vi "PH_uOPA_DelayController.ProcCases.vi"(0 "i ref in":refnum<vi>, 1 "selector":string, 2 "Data":T1, 3 "call cluster":T2={"Object"="", "Selector"="", "CallType"=enum."synchronous", "Async Object"="", "Async Selector"="", "Data Descriptor"="", "Data"=[], "Error #"=0, "Expire"=0}, 5 "error in (no error)":errorcluster) -> (14 "i ref out":refnum<vi>, 17 "answer cluster":T2={"Object"="", "Selector"="", "CallType"=enum."synchronous", "Async Object"="", "Async Selector"="", "Data Descriptor"="", "Data"=[], "Error #"=0, "Expire"=0}, 19 "error out":errorcluster)   [LabVIEW 2014, in "PH_uOPA_DelayController.lvlib"]
doc: "This method is called by a process from within the default case in the event loop. The methods of a class that are linked to events will be called from THIS method. Add your code here."
uses:
  PH_uOPA_DelayController.lvlib
  CS_Core/CSSystem/CoreDefs/CoreDefs.call_type.ctl
  CS_Core/BaseProcess/BaseProcess.descriptor string definition.ctl
  CS_Core/CSSystem/CoreDefs/CoreDefs.rawDataType.ctl
  PH_Basics/PH_StatusHandler/PH_StatusHandler.Status.ctl
  PH_uOPA_DelayController.Limit.ctl
  CS_Core/CSSystem/CoreLib/CoreLib.string 2 byte array.vi
  CS_Core/CSSystem/CoreLib/CoreLib.byte array 2 double.vi
  CS_Core/CSSystem/CoreLib/CoreLib.byte array 2 int.vi
  CS_Core/CSSystem/CoreLib/CoreLib.byte array 2 short.vi
  CS_Core/BaseProcess/BaseProcess.lvlib
  CS_Core/CSSystem/CoreLib/CoreLib.lvlib
  CS_Core/CAEObj/CAEObj.lvlib
  PH_Basics/PH_PSDBWriter/PH_PSDBWriter.lvlib
  PH_Devices/PH_TKTDS-30xx/PH_TKTDS-30xx.lvlib
  PH_Basics/PH_StatusHandler/PH_StatusHandler.lvlib
  PH_Basics/PH_AxisGUI_BaseClass/PH_AxisGUI_BaseClass.lvlib
  PH_Basics/PH_Stepmotor_BaseClass/PH_Stepmotor_BaseClass.lvlib
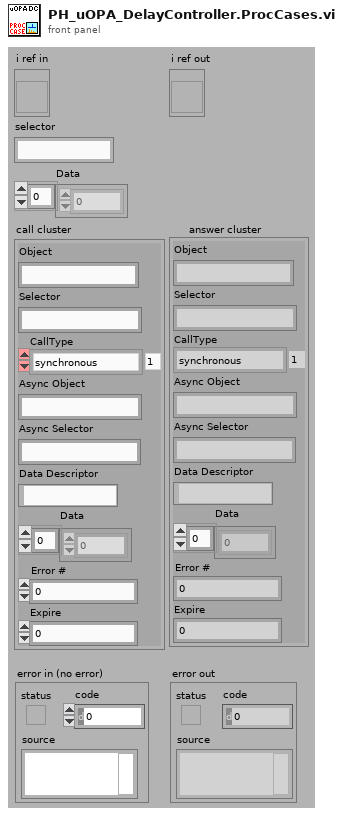
[diagram p1: front panel]
types:
  T1 = typedef "CoreDefs.rawDataType.ctl" = i8[]
  T2 = typedef "CoreDefs.call_type.ctl" = cluster{"Object":string, "Selector":string, "CallType":enum16{"simple", "synchronous", "asynchronous"}, "Async Object":string, "Async Selector":string, "Data Descriptor":T3, "Data":T1, "Error #":i32, "Expire":u32}
  T3 = typedef "BaseProcess.lvlib/BaseProcess.descriptor string definition.ctl" = string
  T4 = typedef "PH_uOPA_DelayController.lvlib/PH_uOPA_DelayController.Limit.ctl" = cluster{"low":dbl, "activate":dbl, "fine":dbl}
  T5 = typedef "PH_StatusHandler.lvlib/PH_StatusHandler.Status.ctl" = i16
  T6 = typedef "PH_PSDBWriter.lvlib/PH_PSDBWriter.PHELIX-Subsystems.ctl" = i32
  T7 = typedef "PH_Stepmotor_BaseClass.lvlib/PH_Stepmotor_BaseClass.Axis Settings.ctl" = cluster{"Sign change":bool, "Width":dbl, "Calibration":dbl, "Unit":string, "Motor Type":T8, "Unit Width":string, "Unit CF":string}
  T8 = typedef "PH_Stepmotor_BaseClass.lvlib/PH_Stepmotor_BaseClass.Motor Type.ctl" = enum16{"Unspecific", "OWIS 49.120.2633", "OWIS 49.060.1033", "OWIS 43.040.2558", "Diamond Motion 2200 series", "OWIS 49.120.266B.MV6", "Calorimeter", "Linear Stage 1", "MICOS VT-80", "MICOS VT-80 S", "Standa Rotstage nt0.95A", "PUF RA 320.200", "PUF RA 800.200", "PUF RA 800.400", "PUF RA 400.50", "1324.nn.800.50", "1324.n9c.800.50", "1324.nn.320.200", "1324.nn.400.200", "1324.nn.800.200", "1324.nn.400.50", "1324.8c9c.800.50", "1324.8c9c.400.200"}
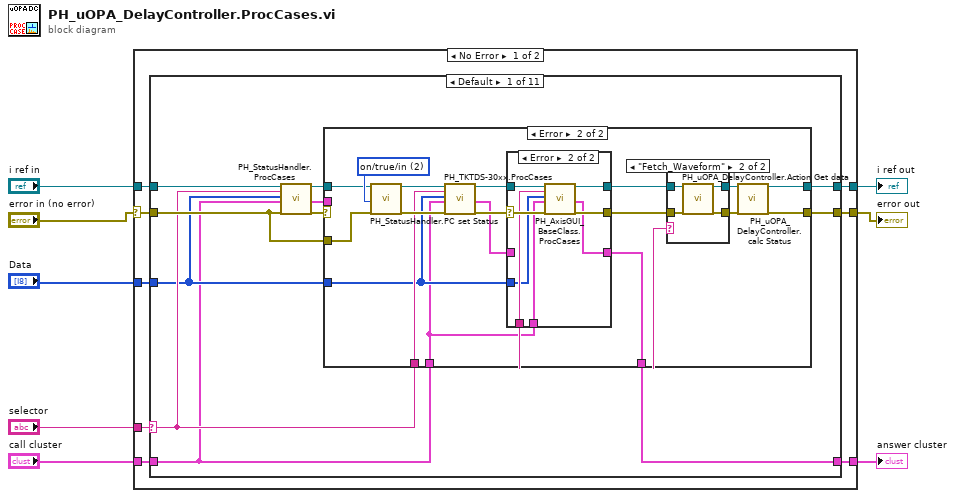
[diagram p0: block diagram]
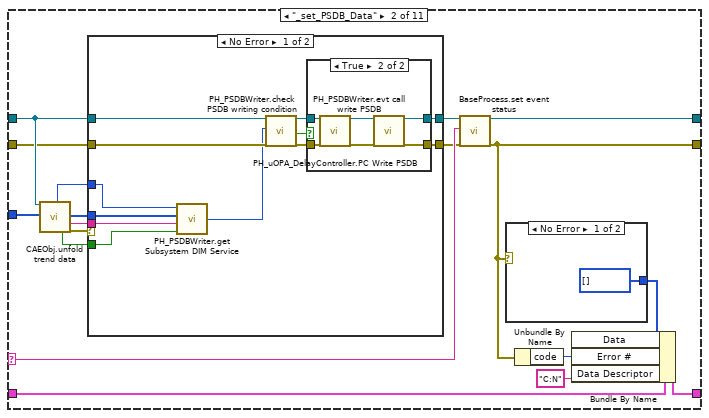
[diagram p5: hidden frame]
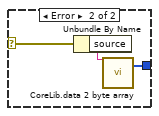
[diagram p8: hidden frame]
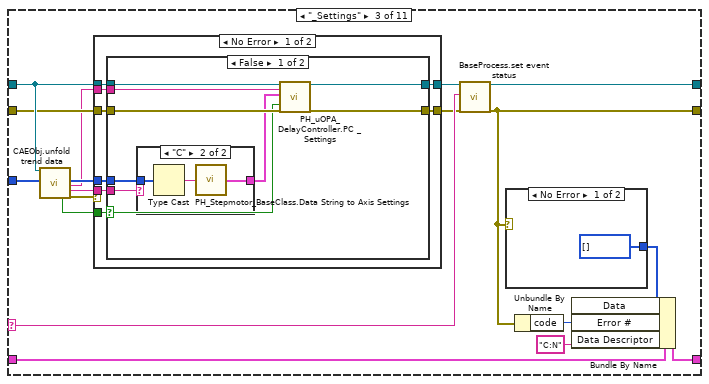
[diagram p9: hidden frame]
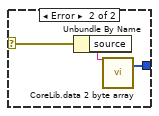
[diagram p13: hidden frame]
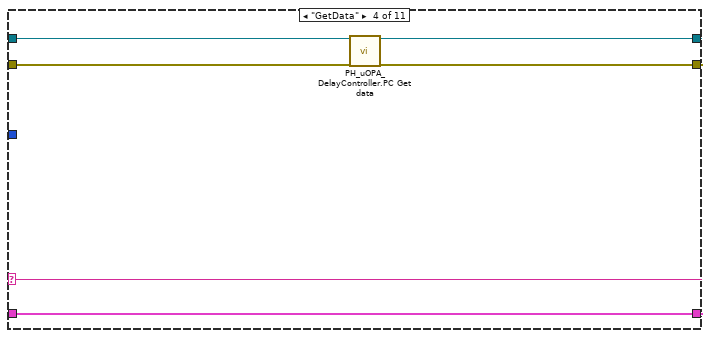
[diagram p14: hidden frame]
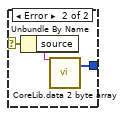
[diagram p15: hidden frame]
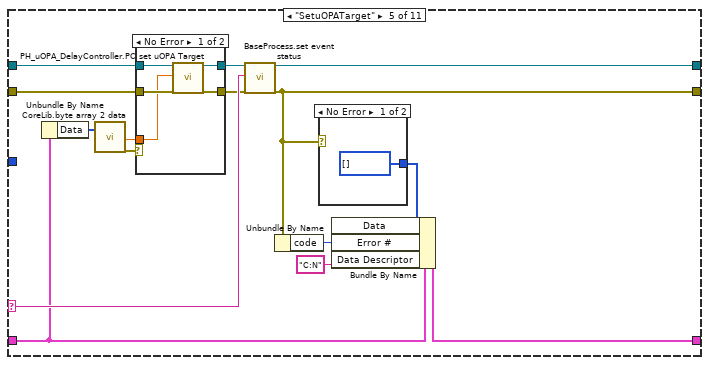
[diagram p16: hidden frame]
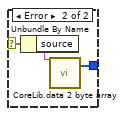
[diagram p18: hidden frame]
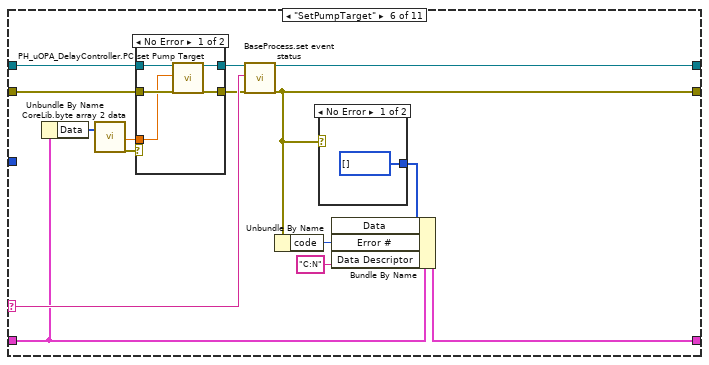
[diagram p19: hidden frame]
diagram:
  n1 = case shown="No Error" "error in (no error)" {
    selector: "error in (no error)" -> [w9 w369]
    tunnel: "selector" -> [w16 _]
    tunnel: [w15 w370] -> w7
    tunnel: "Data" -> [w14 _]
    tunnel: "call cluster" -> [w13 w370]
    tunnel: "i ref in" -> [w12 w371]
    tunnel: [w11 w371] -> w3
    tunnel: [w10 w369] -> w2
    frame No Error {
      n2 = case shown="Default" w16 {
        selector: w16 -> [w19 w78 w122 w161 w181 w207 w233 w259 w287 w316 w348]
        tunnel: w14 -> [w18 w66 w119 _ _ _ _ _ _ _ _]
        tunnel: w12 -> [w24 w70 w118 w159 w176 w202 w228 w254 w282 w311 w343]
        tunnel: [w27 w77 w121 w163 w172 w198 w224 w250 w278 w307 w333] -> w11
        tunnel: w13 -> [w17 w82 w126 w160 w179 w205 w231 w257 w285 w314 w346]
        tunnel: [w25 w81 w125 w166 w185 w211 w237 w263 w291 w320 w352] -> w15
        tunnel: w9 -> [w22 w68 w116 w158 w180 w206 w232 w258 w286 w315 w347]
        tunnel: [w26 w79 w123 w164 w183 w209 w235 w261 w289 w318 w350] -> w10
        frame Default {
          n3 = call "PH_StatusHandler.ProcCases.vi"("i ref in"=w24, "selector"=w19, "Data"=w18, "call cluster"=w17, "error in (no error)"=w22) -> ("i ref out"=w23:refnum<vi>, "answer cluster"=w20:T2, "error out"=w21:errorcluster)  [unwired: 12 in]
          n4 = case shown="Error" w21 {
            selector: w21 -> [w29 _]
            tunnel: [w30 w45] -> w27
            tunnel: [w29 w44] -> w26
            tunnel: w19 -> [_ w37]
            tunnel: w18 -> [_ w36]
            tunnel: w17 -> [_ w35]
            tunnel: [w28 w33] -> w25
            tunnel: w22 -> [_ w32]
            tunnel: w23 -> [w30 w31]
            tunnel: w20 -> [w28 _]
            frame No Error {
            }
            frame Error {
              w48 = T5 2 items=["no info", "off/false/out", "on/true/in", "Failure", "Alarm", "Status 1", "Status 2", "Status 3"] ("Status")
              n5 = call "PH_StatusHandler.PC set Status.vi"("i ref in"=w31, "Status"=w48, "error in (no error)"=w32) -> ("i ref out"=w47:refnum<vi>, "error out"=w46:errorcluster)  [unwired: 15 in]
              n6 = call "PH_TKTDS-30xx.ProcCases.vi"("i ref in"=w47, "selector"=w37, "Data"=w36, "call cluster"=w35, "error in (no error)"=w46) -> ("i ref out"=w40:refnum<vi>, "answer cluster"=w34:T2, "error out"=w38:errorcluster)  [unwired: 12 in]
              n7 = case shown="Error" w38 {
                selector: w38 -> [w50 w56]
                tunnel: [w50 w59] -> w41
                tunnel: w40 -> [w51 w58]
                tunnel: [w51 w57] -> w39
                tunnel: w37 -> [_ w55]
                tunnel: w36 -> [_ w54]
                tunnel: w35 -> [_ w53]
                tunnel: [w49 w52] -> w33
                tunnel: w34 -> [w49 _]
                frame No Error {
                }
                frame Error {
                  n8 = call "PH_AxisGUI_BaseClass.ProcCases.vi"("i ref in"=w58, "selector"=w55, "data"=w54, "call cluster"=w53, "error in"=w56) -> ("i ref out"=w57:refnum<vi>, "answer cluster"=w52:T2, "error out"=w59:errorcluster)  [unwired: 12 in]
                }
              }
              n9 = case shown="\"Fetch_Waveform\"" w37 {
                tunnel: w39 -> [w61 w65]
                tunnel: [w61 w64] -> w43
                tunnel: w41 -> [w60 w63]
                tunnel: [w60 w62] -> w42
                frame Default {
                }
                frame "Fetch_Waveform" {
                  n10 = call "PH_uOPA_DelayController.Action Get data.vi"("i ref in"=w65, "error IO"=w63) -> ("i ref out"=w64:refnum<vi>, "error out"=w62:errorcluster)  [unwired: 16 in]
                }
              }
              n11 = call "PH_uOPA_DelayController.calc Status.vi"("i ref in"=w43, "error in"=w42) -> ("i ref out"=w45:refnum<vi>, "error out"=w44:errorcluster)  [unwired: 16 in]
            }
          }
        }
        frame "_set_PSDB_Data" {
          n12 = call "CAEObj.unfold trend data.vi"("i ref in"=w70, "raw trend data"=w66) -> ("quality"=w71:i32, "no link"=w74:bool, "data"=w72:i8[], "typeDescriptor"=w73:string, "error out"=w75:errorcluster)  [unwired: 9 in, 4 out]
          n13 = case shown="No Error" w75 {
            tunnel: w68 -> [w95 w105]
            tunnel: [w94 w104] -> w69
            tunnel: [w93 w105] -> w67
            tunnel: w70 -> [w91 w104]
            tunnel: w74 -> [w86 _]
            tunnel: w73 -> [w87 _]
            tunnel: w72 -> [w88 _]
            tunnel: w71 -> [w85 _]
            frame No Error {
              n14 = call "PH_PSDBWriter.get Subsystem DIM Service.vi"("no link"=w86, "typeDescriptor"=w87, "data"=w88, "quality"=w85) -> ("PHELIX Subsystems"=w84:T6)
              n15 = call "PH_PSDBWriter.check PSDB writing condition.vi"("i ref in"=w91, "wanted Subsystem"=w84, "error IO"=w95) -> ("i ref out"=w90:refnum<vi>, "write PSDB?"=w89:bool, "error out"=w92:errorcluster)  [unwired: 14 in]
              n16 = case shown="True" w89 {
                tunnel: w92 -> [w96 w103]
                tunnel: [w97 w100] -> w94
                tunnel: [w96 w98] -> w93
                tunnel: w90 -> [w97 w102]
                frame False {
                }
                frame True {
                  n17 = call "PH_uOPA_DelayController.PC Write PSDB.vi"("i ref in"=w102, "error IO"=w103) -> ("i ref out"=w101:refnum<vi>, "error out"=w99:errorcluster)  [unwired: 16 in]
                  n18 = call "PH_PSDBWriter.evt call write PSDB.vi"("i ref in"=w101, "error in (no error)"=w99) -> ("i ref out"=w100:refnum<vi>, "error out"=w98:errorcluster)  [unwired: 16 in]
                }
              }
            }
            frame Error {
            }
          }
          n19 = call "BaseProcess.set event status.vi"("i ref in"=w69, "EventStatus"=w78, "error in (no error)"=w67) -> ("i ref out"=w77:refnum<vi>, "error out"=w79:errorcluster)  [unwired: 14 in, 1 out]
          n20 = case shown="No Error" w79 {
            selector: w79 -> [_ w109]
            tunnel: [T1 [] ("byteArray out") w108] -> w80
            frame No Error {
            }
            frame Error {
              n21 = Unbundle By Name(w109) -> ("source"=w107:string)
              n22 = call-poly "CoreLib.data 2 byte array.vi"("string"=w107) -> ("byteArray out"=w108:T1)  [unwired: 18 in]
            }
          }
          n23 = Unbundle By Name(w79) -> ("code"=w83:i32)
          n24 = Bundle By Name(cluster=w82, "Data"=w80, "Error #"=w83, "Data Descriptor"="C:N") -> (w81:T2)
        }
        frame "_Settings" {
          n25 = call "CAEObj.unfold trend data.vi"("i ref in"=w118, "raw trend data"=w119) -> ("no link"=w111:bool, "data"=w114:i8[], "serviceName"=w113:string, "typeDescriptor"=w110:string, "error out"=w112:errorcluster)  [unwired: 9 in, 4 out]
          n26 = case shown="No Error" w112 {
            tunnel: w114 -> [w130 _]
            tunnel: w118 -> [w134 w151]
            tunnel: [w133 w151] -> w117
            tunnel: w116 -> [w135 w150]
            tunnel: [w132 w150] -> w115
            tunnel: w111 -> [w131 _]
            tunnel: w110 -> [w129 _]
            tunnel: w113 -> [w128 _]
            frame No Error {
              n27 = case "NO LINK?" shown="False" w131 {
                selector: w131 -> [w141 _]
                tunnel: w135 -> [w143 w149]
                tunnel: w134 -> [w144 w148]
                tunnel: [w139 w148] -> w133
                tunnel: [w140 w149] -> w132
                tunnel: w129 -> [w137 _]
                tunnel: w130 -> [w138 _]
                tunnel: w128 -> [w142 _]
                frame False {
                  n28 = case shown="\"C\"" w137 {
                    tunnel: [_ w145] -> w136
                    tunnel: w138 -> [_ w147]
                    frame Default {
                    }
                    frame "C" {
                      n29 = Type Cast(x=w147) -> (*(type *) &x=w146:string)  [unwired: 1 in]
                      n30 = call "PH_Stepmotor_BaseClass.Data String to Axis Settings.vi"("Data String"=w146) -> ("Axis Settings"=w145:T7)  [unwired: 1 out]
                    }
                  }
                  n31 = call "PH_uOPA_DelayController.PC _Settings.vi"("VI in"=w144, "serviceName"=w142, "Axis Settings"=w136, "no link"=w141, "error in (no error)"=w143) -> ("VI out"=w139:refnum<vi>, "error out"=w140:errorcluster)  [unwired: 13 in]
                }
                frame True {
                }
              }
            }
            frame Error {
            }
          }
          n32 = call "BaseProcess.set event status.vi"("i ref in"=w117, "EventStatus"=w122, "error in (no error)"=w115) -> ("i ref out"=w121:refnum<vi>, "error out"=w123:errorcluster)  [unwired: 14 in, 1 out]
          n33 = case shown="No Error" w123 {
            selector: w123 -> [_ w155]
            tunnel: [T1 [] ("byteArray out") w154] -> w124
            frame No Error {
            }
            frame Error {
              n34 = Unbundle By Name(w155) -> ("source"=w153:string)
              n35 = call-poly "CoreLib.data 2 byte array.vi"("string"=w153) -> ("byteArray out"=w154:T1)  [unwired: 18 in]
            }
          }
          n36 = Unbundle By Name(w123) -> ("code"=w127:i32)
          n37 = Bundle By Name(cluster=w126, "Data"=w124, "Error #"=w127, "Data Descriptor"="C:N") -> (w125:T2)
        }
        frame "GetData" {
          n38 = call "PH_uOPA_DelayController.PC Get data.vi"("i ref in"=w159, "error IO"=w158) -> ("i ref out"=w157:refnum<vi>, "error out"=w156:errorcluster)  [unwired: 16 in]
          n39 = call "BaseProcess.set event status.vi"("i ref in"=w157, "EventStatus"=w161, "error in (no error)"=w156) -> ("i ref out"=w163:refnum<vi>, "error out"=w164:errorcluster)  [unwired: 14 in, 1 out]
          n40 = Unbundle By Name(w164) -> ("code"=w167:i32)
          n41 = case shown="No Error" w164 {
            selector: w164 -> [_ w171]
            tunnel: [T1 [] ("byteArray out") w170] -> w165
            frame No Error {
            }
            frame Error {
              n42 = Unbundle By Name(w171) -> ("source"=w169:string)
              n43 = call-poly "CoreLib.data 2 byte array.vi"("string"=w169) -> ("byteArray out"=w170:T1)  [unwired: 18 in]
            }
          }
          n44 = Bundle By Name(cluster=w160, "Data"=w165, "Error #"=w167, "Data Descriptor"="C:N") -> (w166:T2)
        }
        frame "SetuOPATarget" {
          n45 = Unbundle By Name(w179) -> ("Data"=w178:T1)
          n46 = call-poly "CoreLib.byte array 2 data.vi"("byteArray"=w178) -> ("d64"=w175:dbl, "error out"=w174:errorcluster)  [unwired: 16 in, 1 out]
          n47 = case shown="No Error" w174 {
            tunnel: w180 -> [w191 w192]
            tunnel: [w190 w192] -> w177
            tunnel: [w189 w193] -> w173
            tunnel: w176 -> [w188 w193]
            tunnel: w175 -> [w187 _]
            frame No Error {
              n48 = call "PH_uOPA_DelayController.PC set uOPA Target.vi"("VI in"=w188, "uOPA Target"=w187, "error in (no error)"=w191) -> ("VI out"=w189:refnum<vi>, "error out"=w190:errorcluster)  [unwired: 15 in]
            }
            frame Error {
            }
          }
          n49 = call "BaseProcess.set event status.vi"("i ref in"=w173, "EventStatus"=w181, "error in (no error)"=w177) -> ("i ref out"=w172:refnum<vi>, "error out"=w183:errorcluster)  [unwired: 14 in, 1 out]
          n50 = Unbundle By Name(w183) -> ("code"=w186:i32)
          n51 = case shown="No Error" w183 {
            selector: w183 -> [_ w197]
            tunnel: [T1 [] ("byteArray out") w196] -> w184
            frame No Error {
            }
            frame Error {
              n52 = Unbundle By Name(w197) -> ("source"=w195:string)
              n53 = call-poly "CoreLib.data 2 byte array.vi"("string"=w195) -> ("byteArray out"=w196:T1)  [unwired: 18 in]
            }
          }
          n54 = Bundle By Name(cluster=w179, "Data"=w184, "Error #"=w186, "Data Descriptor"="C:N") -> (w185:T2)
        }
        frame "SetPumpTarget" {
          n55 = Unbundle By Name(w205) -> ("Data"=w204:T1)
          n56 = call-poly "CoreLib.byte array 2 data.vi"("byteArray"=w204) -> ("d64"=w201:dbl, "error out"=w200:errorcluster)  [unwired: 16 in, 1 out]
          n57 = case shown="No Error" w200 {
            tunnel: w206 -> [w217 w218]
            tunnel: [w216 w218] -> w203
            tunnel: [w215 w219] -> w199
            tunnel: w202 -> [w214 w219]
            tunnel: w201 -> [w213 _]
            frame No Error {
              n58 = call "PH_uOPA_DelayController.PC set Pump Target.vi"("VI in"=w214, "Pump Target"=w213, "error in (no error)"=w217) -> ("VI out"=w215:refnum<vi>, "error out"=w216:errorcluster)  [unwired: 15 in]
            }
            frame Error {
            }
          }
          n59 = call "BaseProcess.set event status.vi"("i ref in"=w199, "EventStatus"=w207, "error in (no error)"=w203) -> ("i ref out"=w198:refnum<vi>, "error out"=w209:errorcluster)  [unwired: 14 in, 1 out]
          n60 = Unbundle By Name(w209) -> ("code"=w212:i32)
          n61 = case shown="No Error" w209 {
            selector: w209 -> [_ w223]
            tunnel: [T1 [] ("byteArray out") w222] -> w210
            frame No Error {
            }
            frame Error {
              n62 = Unbundle By Name(w223) -> ("source"=w221:string)
              n63 = call-poly "CoreLib.data 2 byte array.vi"("string"=w221) -> ("byteArray out"=w222:T1)  [unwired: 18 in]
            }
          }
          n64 = Bundle By Name(cluster=w205, "Data"=w210, "Error #"=w212, "Data Descriptor"="C:N") -> (w211:T2)
        }
        frame "SetPumpLimit" {
          n65 = Unbundle By Name(w231) -> ("Data"=w230:T1)
          n66 = call-poly "CoreLib.byte array 2 data.vi"("byteArray"=w230) -> ("d64"=w227:dbl, "error out"=w226:errorcluster)  [unwired: 16 in, 1 out]
          n67 = case shown="No Error" w226 {
            tunnel: w232 -> [w243 w244]
            tunnel: [w242 w244] -> w229
            tunnel: [w241 w245] -> w225
            tunnel: w228 -> [w240 w245]
            tunnel: w227 -> [w239 _]
            frame No Error {
              n68 = call "PH_uOPA_DelayController.PC set Pump Limit.vi"("VI in"=w240, "Pump Limit [%]"=w239, "error in (no error)"=w243) -> ("VI out"=w241:refnum<vi>, "error out"=w242:errorcluster)  [unwired: 15 in]
            }
            frame Error {
            }
          }
          n69 = call "BaseProcess.set event status.vi"("i ref in"=w225, "EventStatus"=w233, "error in (no error)"=w229) -> ("i ref out"=w224:refnum<vi>, "error out"=w235:errorcluster)  [unwired: 14 in, 1 out]
          n70 = Unbundle By Name(w235) -> ("code"=w238:i32)
          n71 = case shown="No Error" w235 {
            selector: w235 -> [_ w249]
            tunnel: [T1 [] ("byteArray out") w248] -> w236
            frame No Error {
            }
            frame Error {
              n72 = Unbundle By Name(w249) -> ("source"=w247:string)
              n73 = call-poly "CoreLib.data 2 byte array.vi"("string"=w247) -> ("byteArray out"=w248:T1)  [unwired: 18 in]
            }
          }
          n74 = Bundle By Name(cluster=w231, "Data"=w236, "Error #"=w238, "Data Descriptor"="C:N") -> (w237:T2)
        }
        frame "SetSampleLength" {
          n75 = Unbundle By Name(w257) -> ("Data"=w256:T1)
          n76 = call-poly "CoreLib.byte array 2 data.vi"("byteArray"=w256) -> ("i32"=w253:i32, "error out"=w252:errorcluster)  [unwired: 16 in, 1 out]
          n77 = case shown="No Error" w252 {
            tunnel: w258 -> [w271 w272]
            tunnel: [w267 w272] -> w255
            tunnel: [w265 w273] -> w251
            tunnel: w254 -> [w269 w273]
            tunnel: w253 -> [w268 _]
            frame No Error {
              n78 = call "PH_uOPA_DelayController.PC set Sample Length.vi"("VI in"=w269, "Sample Length"=w268, "error in (no error)"=w271) -> ("VI out"=w266:refnum<vi>, "error out"=w270:errorcluster)  [unwired: 15 in]
              n79 = call "PH_uOPA_DelayController.set Initialize Mean.vi"("VI in"=w266, "error in (no error)"=w270) -> ("VI out"=w265:refnum<vi>, "error out"=w267:errorcluster)  [unwired: 16 in]
            }
            frame Error {
            }
          }
          n80 = call "BaseProcess.set event status.vi"("i ref in"=w251, "EventStatus"=w259, "error in (no error)"=w255) -> ("i ref out"=w250:refnum<vi>, "error out"=w261:errorcluster)  [unwired: 14 in, 1 out]
          n81 = Unbundle By Name(w261) -> ("code"=w264:i32)
          n82 = case shown="No Error" w261 {
            selector: w261 -> [_ w277]
            tunnel: [T1 [] ("byteArray out") w276] -> w262
            frame No Error {
            }
            frame Error {
              n83 = Unbundle By Name(w277) -> ("source"=w275:string)
              n84 = call-poly "CoreLib.data 2 byte array.vi"("string"=w275) -> ("byteArray out"=w276:T1)  [unwired: 18 in]
            }
          }
          n85 = Bundle By Name(cluster=w257, "Data"=w262, "Error #"=w264, "Data Descriptor"="C:N") -> (w263:T2)
        }
        frame "SetFeedbackControl" {
          n86 = Unbundle By Name(w285) -> ("Data"=w284:T1)
          n87 = call-poly "CoreLib.byte array 2 data.vi"("byteArray"=w284) -> ("i16"=w281:i16, "error out"=w280:errorcluster)  [unwired: 16 in, 1 out]
          n88 = case shown="No Error" w280 {
            tunnel: w286 -> [w300 w301]
            tunnel: [w293 w301] -> w283
            tunnel: [w295 w302] -> w279
            tunnel: w282 -> [w299 w302]
            tunnel: w281 -> [w298 _]
            frame No Error {
              n89 = Greater Than 0?(x=w298) -> (x > 0?=w297:bool)
              n90 = call "PH_uOPA_DelayController.PC set Feedback Control.vi"("VI in"=w299, "Feedback Control"=w297, "error in (no error)"=w300) -> ("VI out"=w296:refnum<vi>, "error out"=w294:errorcluster)  [unwired: 15 in]
              n91 = call "PH_uOPA_DelayController.set Initialize Mean.vi"("VI in"=w296, "error in (no error)"=w294) -> ("VI out"=w295:refnum<vi>, "error out"=w293:errorcluster)  [unwired: 16 in]
            }
            frame Error {
            }
          }
          n92 = call "BaseProcess.set event status.vi"("i ref in"=w279, "EventStatus"=w287, "error in (no error)"=w283) -> ("i ref out"=w278:refnum<vi>, "error out"=w289:errorcluster)  [unwired: 14 in, 1 out]
          n93 = Unbundle By Name(w289) -> ("code"=w292:i32)
          n94 = case shown="No Error" w289 {
            selector: w289 -> [_ w306]
            tunnel: [T1 [] ("byteArray out") w305] -> w290
            frame No Error {
            }
            frame Error {
              n95 = Unbundle By Name(w306) -> ("source"=w304:string)
              n96 = call-poly "CoreLib.data 2 byte array.vi"("string"=w304) -> ("byteArray out"=w305:T1)  [unwired: 18 in]
            }
          }
          n97 = Bundle By Name(cluster=w285, "Data"=w290, "Error #"=w292, "Data Descriptor"="C:N") -> (w291:T2)
        }
        frame "SetWidthwhileFeedback" {
          n98 = Unbundle By Name(w314) -> ("Data"=w313:T1)
          n99 = call-poly "CoreLib.byte array 2 data.vi"("byteArray"=w313) -> ("d64"=w310:dbl, "error out"=w309:errorcluster)  [unwired: 16 in, 1 out]
          n100 = case shown="No Error" w309 {
            tunnel: w315 -> [w326 w327]
            tunnel: [w323 w327] -> w312
            tunnel: [w324 w328] -> w308
            tunnel: w311 -> [w325 w328]
            tunnel: w310 -> [w322 _]
            frame No Error {
              n101 = call "PH_uOPA_DelayController.PC set Width while Feedback.vi"("VI in"=w325, "Width while Feedback"=w322, "error in (no error)"=w326) -> ("VI out"=w324:refnum<vi>, "error out"=w323:errorcluster)  [unwired: 15 in]
            }
            frame Error {
            }
          }
          n102 = call "BaseProcess.set event status.vi"("i ref in"=w308, "EventStatus"=w316, "error in (no error)"=w312) -> ("i ref out"=w307:refnum<vi>, "error out"=w318:errorcluster)  [unwired: 14 in, 1 out]
          n103 = Unbundle By Name(w318) -> ("code"=w321:i32)
          n104 = case shown="No Error" w318 {
            selector: w318 -> [_ w332]
            tunnel: [T1 [] ("byteArray out") w331] -> w319
            frame No Error {
            }
            frame Error {
              n105 = Unbundle By Name(w332) -> ("source"=w330:string)
              n106 = call-poly "CoreLib.data 2 byte array.vi"("string"=w330) -> ("byteArray out"=w331:T1)  [unwired: 18 in]
            }
          }
          n107 = Bundle By Name(cluster=w314, "Data"=w319, "Error #"=w321, "Data Descriptor"="C:N") -> (w320:T2)
        }
        frame "SetuOPALimits" {
          n108 = Unbundle By Name(w346) -> ("Data"=w345:T1)
          n109 = call-poly "CoreLib.byte array 2 data.vi"("byteArray"=w345) -> ("byteArray out"=w336:T1, "d64"=w342:dbl, "error out"=w340:errorcluster)  [unwired: 16 in]
          n110 = call-poly "CoreLib.byte array 2 data.vi"("byteArray"=w336, "error in (no error)"=w340) -> ("byteArray out"=w335:T1, "d64"=w338:dbl, "error out"=w341:errorcluster)  [unwired: 15 in]
          n111 = call-poly "CoreLib.byte array 2 data.vi"("byteArray"=w335, "error in (no error)"=w341) -> ("d64"=w337:dbl, "error out"=w339:errorcluster)  [unwired: 15 in, 1 out]
          n112 = case shown="No Error" w339 {
            tunnel: w347 -> [w362 w363]
            tunnel: [w361 w363] -> w344
            tunnel: [w360 w364] -> w334
            tunnel: w343 -> [w359 w364]
            tunnel: w342 -> [w356 _]
            tunnel: w338 -> [w355 _]
            tunnel: w337 -> [w354 _]
            frame No Error {
              n113 = Bundle By Name(cluster=T4 {"low"=20.0, "activate"=75.0, "fine"=95.0} ("Limits"), "low"=w356, "activate"=w355, "fine"=w354) -> (w357:T4)
              n114 = call "PH_uOPA_DelayController.PC set uOPA Limits.vi"("VI in"=w359, "Limits"=w357, "error in (no error)"=w362) -> ("VI out"=w360:refnum<vi>, "error out"=w361:errorcluster)  [unwired: 15 in]
            }
            frame Error {
            }
          }
          n115 = call "BaseProcess.set event status.vi"("i ref in"=w334, "EventStatus"=w348, "error in (no error)"=w344) -> ("i ref out"=w333:refnum<vi>, "error out"=w350:errorcluster)  [unwired: 14 in, 1 out]
          n116 = Unbundle By Name(w350) -> ("code"=w353:i32)
          n117 = case shown="No Error" w350 {
            selector: w350 -> [_ w368]
            tunnel: [T1 [] ("byteArray out") w367] -> w351
            frame No Error {
            }
            frame Error {
              n118 = Unbundle By Name(w368) -> ("source"=w366:string)
              n119 = call-poly "CoreLib.data 2 byte array.vi"("string"=w366) -> ("byteArray out"=w367:T1)  [unwired: 18 in]
            }
          }
          n120 = Bundle By Name(cluster=w346, "Data"=w351, "Error #"=w353, "Data Descriptor"="C:N") -> (w352:T2)
        }
      }
    }
    frame Error {
    }
  }
  "answer cluster" <- w7
  "i ref out" <- w3
  "error out" <- w2
